vi "IV.vi"(1 "Wait for continue":bool, 2 "Run uninterrupted?":bool, 3 "Device Category IN:":string(combo)="Short Strip" caption="Device Category:", 4 "Batch No. IN:":string caption="Batch No.:", 5 "Wafer No. IN:":string caption="Wafer:", 6 "DB Serial No. IN:":string caption="DB Serial No.:") -> (0 "Done!":bool)   [LabVIEW 2018]
doc: "Performs IV measurements according to ATLAS ITk Quality Control Specifications."
uses:
  general_VIs/globals/QC_MeasurementSetup.vi
  general_VIs/globals/QC_RunInformation.vi
  InstrControl/InstrumentSetup.vi
  InstrControl/Switching/Switching.lvclass
  InstrControl/SupplyControl/SupplyControl.lvclass
  InstrControl/ArduinoControl/ArduinoControl.lvclass
  InstrControl/InstrControl.lvclass
panel:
  out "Tab Control 2":enum32{"IV Setup", "IV Scan"}(tab)
  in  "V_breakdown limit [V]":dbl=-500.0
  in  "Set current limit?":bool
  in  "Current Limit [µA]":dbl=1.0 min=0.0001 format="%.3f"
  in  "Measurement Configurations":bool
  in  "hold steps IN":i32=6 caption="hold steps"
  in  "Initial volts [V] IN":dbl caption="Initial volts [V]"
  in  "Final volts [V] IN":dbl=-700.0 caption="Final volts [V]"
  in  "step [V] IN":dbl=10.0 caption="step [V]" format="%.1f"
  in  "step interval [s] IN":i32=10 caption="step interval [s]"
  in  "Continue":bool
  in  "Quit":bool
  out "hold steps":i32=6
  out "RH":dbl[](array[numeric]) caption="RH [%]" format="%#.2f"
  out "Temp.":dbl[](array[numeric]) caption="Temp. [°C]" format="%#.2f"
  out "Current":dbl[](array[numeric]) caption="Current [nA]"
  out "Volts":dbl[](array[numeric]) caption="Volts [V]"
  out "step interval [s]":i32=10
  out "step [V]":dbl=10.0 format="%.1f"
  out "Final volts [V]":dbl=-700.0 format="%.1f"
  out "Initial volts [V]":dbl format="%.1f"
  out "Igraph":cluster{dbl[], dbl[]}(graph)
  in  "Scales":T1(ring)
  in  "Iscale":enum16{"nanoAmps", "microAmps", "milliAmps"}(ring)
  out "positive ramp?":bool
  out "Tab Control":enum32{"IV Setup", "IV Scan"}(tab)
  in  "Comments":string caption="Comments:"
  in  "Auto save files":bool=TRUE
  in  "Hardware Configurations":bool
  in  "User:":string(combo)="Vera"
  in  "IV Supply":string(combo)="Keithley 2410"
  in  "Temperature":enum16{"Read Arduino", "Enter manually"}(ring)
  in  "Manufacturer:":string(combo)="Hamamatsu"
  in  "abort":bool
  out "Device Category:":string
  out "DB Serial No.:":string
  out "Current Volts:":dbl format="%.2f"
  in  "quit (no save)":bool
  in  "Quit & Save":bool
  out "Bias On/Off:":bool
  out "STATUS 1":string
  out "Initiated:":string
  out "Wafer:":string
  out "No of steps":u32
  out "Current reading No.":u32
  out "Last reading at:":string
  # "University of\nCambridge"
  # "Strip Sensor QC: IV"
  # "Vertical Scale:"
  # "Measurement Configuration"
  # "IV Scan parameters:"
  # "Last 5 readings:"
  # "n-4"
  # "n-3"
  # "n-2"
  # "n-1"
  # "n"
  # "DUT Description"
  # "Hardware"
  # "DUT & Test Description:"
  # "Current status:"
  # "Rdg No:"
  # "out of"
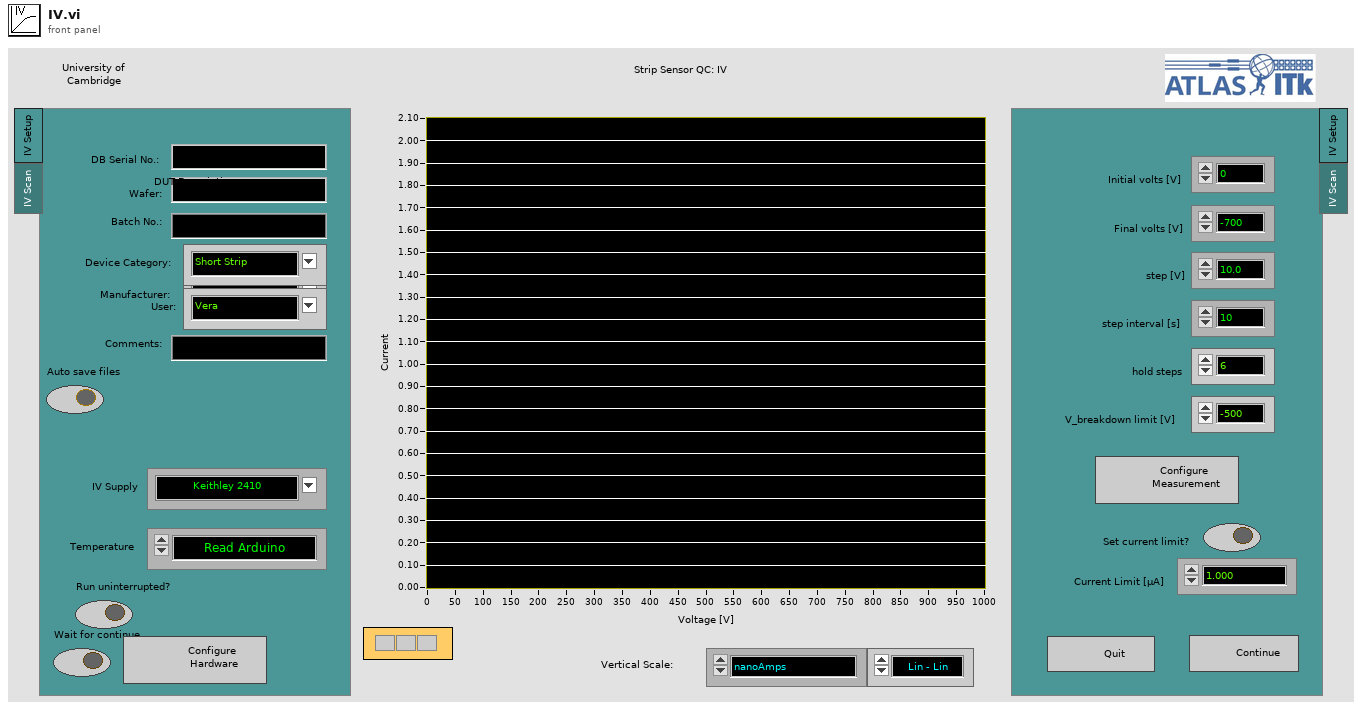
[diagram p1: front panel]
types:
  T1 = enum16{"Lin - Lin", "Log - Lin", "Lin - Log", "Log - log"}
  T2 = enum16{"Supply", "LCR", "Multimeter", "Switching"}
  T3 = enum16{"Reset", "Read Array", "Read Element", "Write Element", "Write Array", "Add Element", "Add Array"}
  T4 = enum16{"Reset", "Ground", "Striptest SMU", "Striptest LCR", "IV", "CV", "Interstrip Cap", "Interstrip Res"}
  T5 = enum32{"IV", "CV", "Stability", "Striptest", "Cis", "Ris", "PTP"}
  T6 = cluster{"Sensor Serial No.:":string, "Wafer:":string, "Batch:":string, "Manufacturer:":string, "Device Category:":string, "Database Serial No.:":string, "Date Initiated:":string, "Time Initiated:":string, "Test":string, "Probeplan used:":string, "End of Run comment:":string, "User:":string, "Vbias SMU":string, "LCR":string, "Test SMU":string, "Test DMM":string, "Comments":string}
  T7 = cluster{"Institute":string, "Manufacturers":string[], "Devices":string[], "Serialnumbers Lookup DB":string, "Data directory":string, "Backup & screenshot directory":string, "List of known users":string[], "Measurement switch not used":bool, "Measurement Switch":string, "DUT Switch":string, "Rseries IV [MOhm]":string, "Rshunt IV [MOhm]":string, "Rseries CV [MOhm]":string, "DC blocking Cap [µF]":string, "Rseries LCR [MOhm]":string, "Rseries stability [MOhm]":string, "Rshunt stability [MOhm]":string, "Rseries striptest bias [MOhm]":string, "Rseries strip pinhole [MOhm]":string}
  T8 = cluster{"Supply":refnum<class "SupplyControl.lvclass">, "Arduino":refnum<class "ArduinoControl.lvclass">, "Measurement switch":refnum<class "Switching.lvclass">, "Initial Voltage [V]":dbl, "Final Voltage [V]":dbl, "Step Size [V]":dbl, "Step Interval [s]":i32, "Number Of Steps":u32, "Ramp down steps [V]":dbl, "Ramp down Interval [s]":i32, "hold steps":i32, "Set Current Limit?":bool, "Current Limit [µA]":dbl, "Temperature Readout":enum16{"Read Arduino", "Enter manually"}, "Supply Name":string, "V_breakdown Limit [V]":dbl, "Measurement switch used?":bool}
  T9 = cluster{"VISA address":refnum<visa-resource-name>, "T sensor":enum16{"SHT", "DS"}, "Arduino":refnum<class "ArduinoControl.lvclass">}
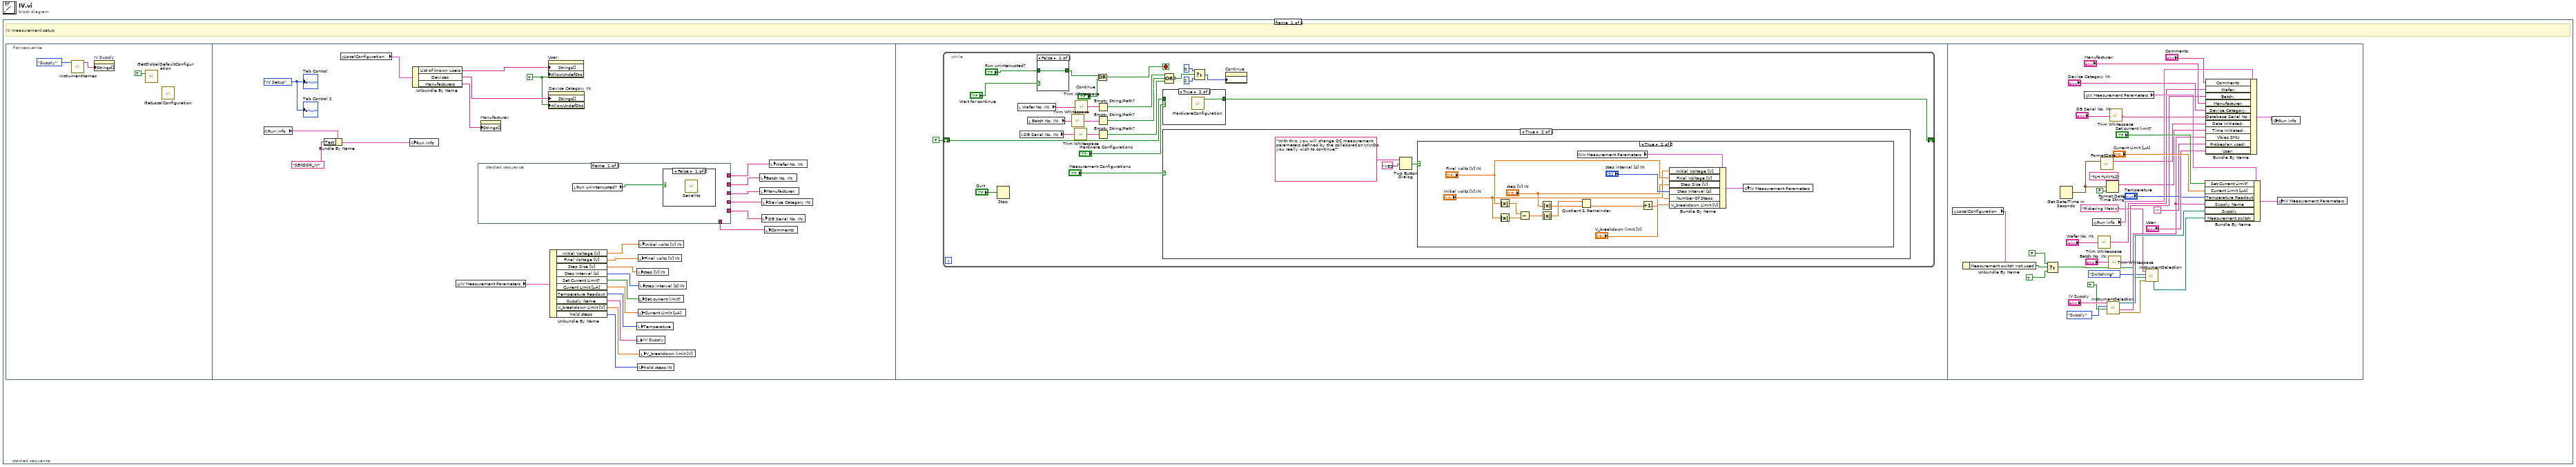
[diagram p0: block diagram]
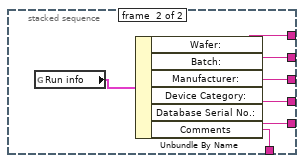
[diagram p3: hidden frame]
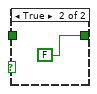
[diagram p4: hidden frame]
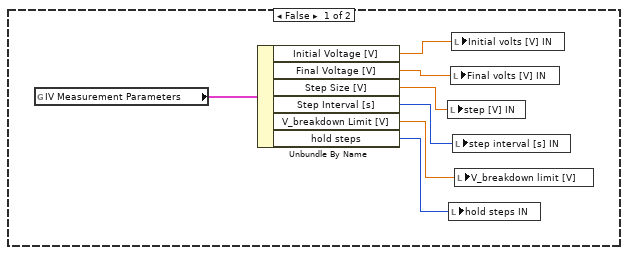
[diagram p6: hidden frame]
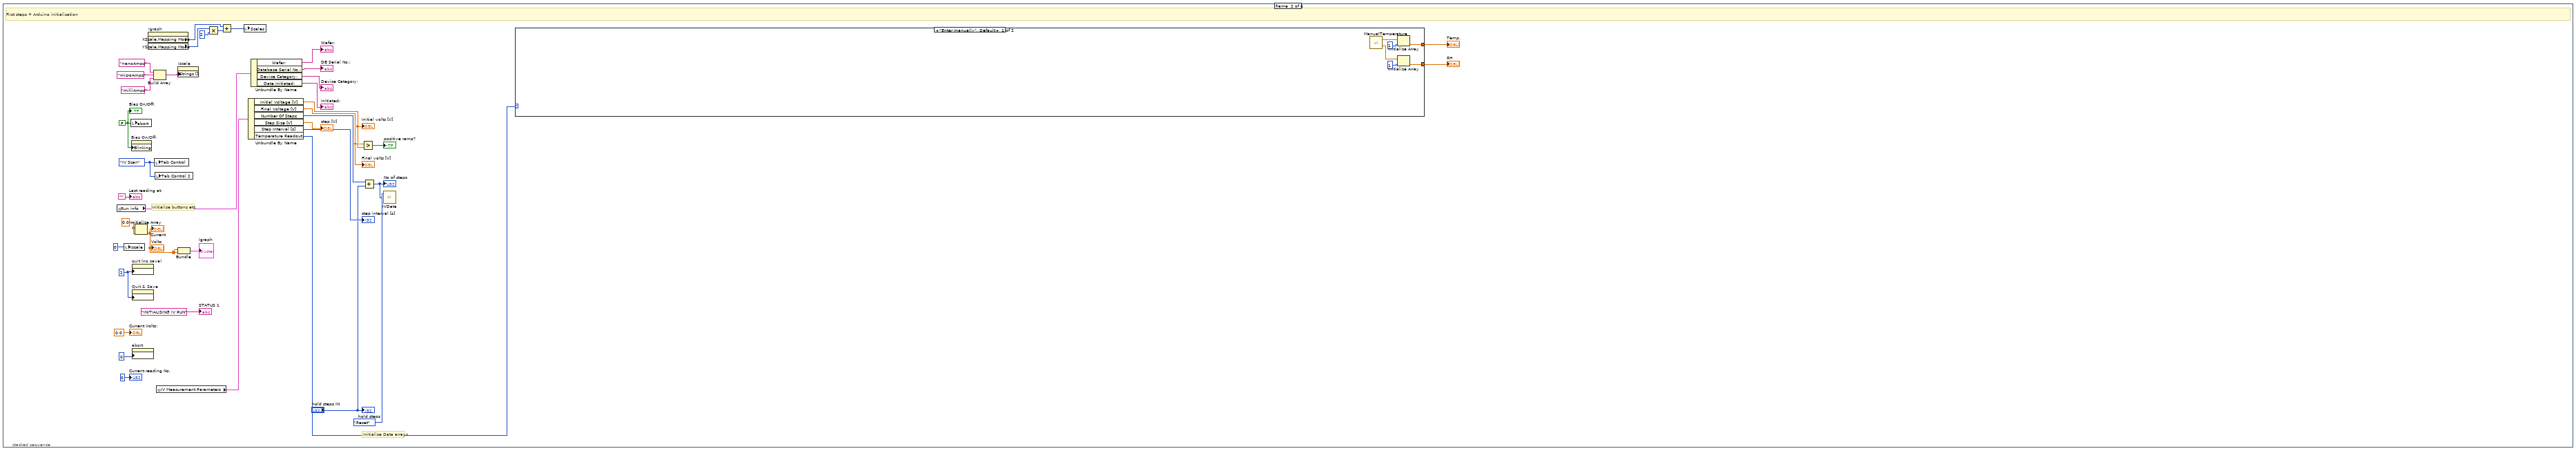
[diagram p8: hidden frame]
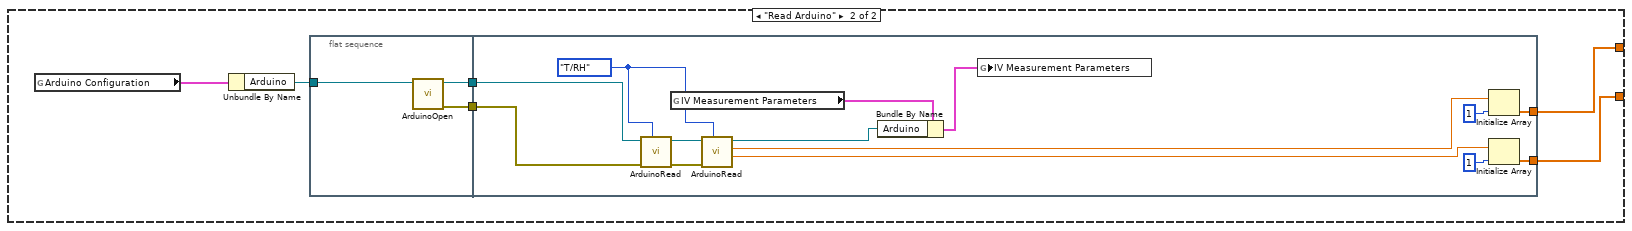
[diagram p9: hidden frame]
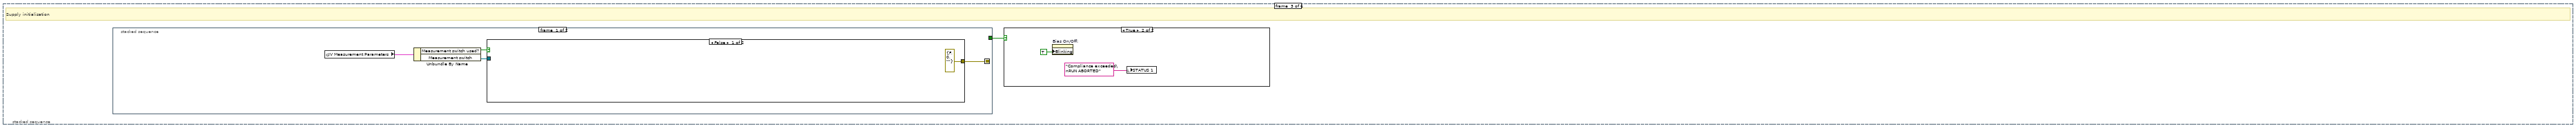
[diagram p10: hidden frame]
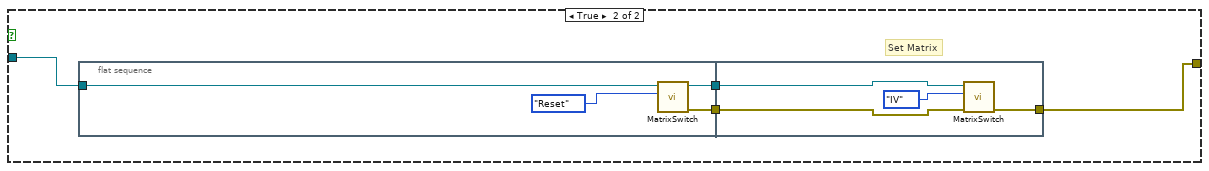
[diagram p11: hidden frame]
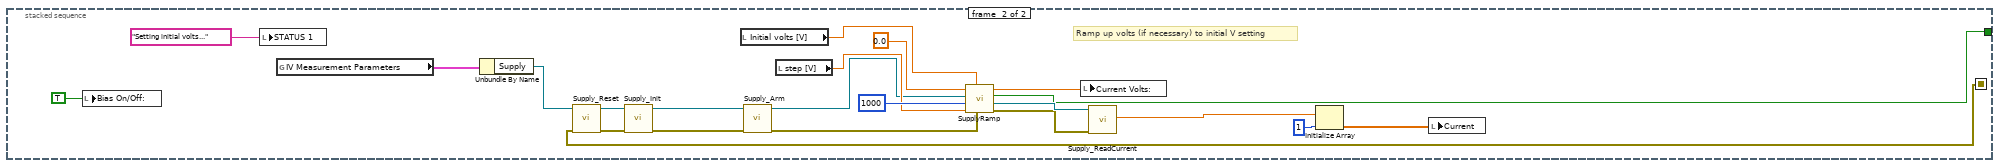
[diagram p12: hidden frame]
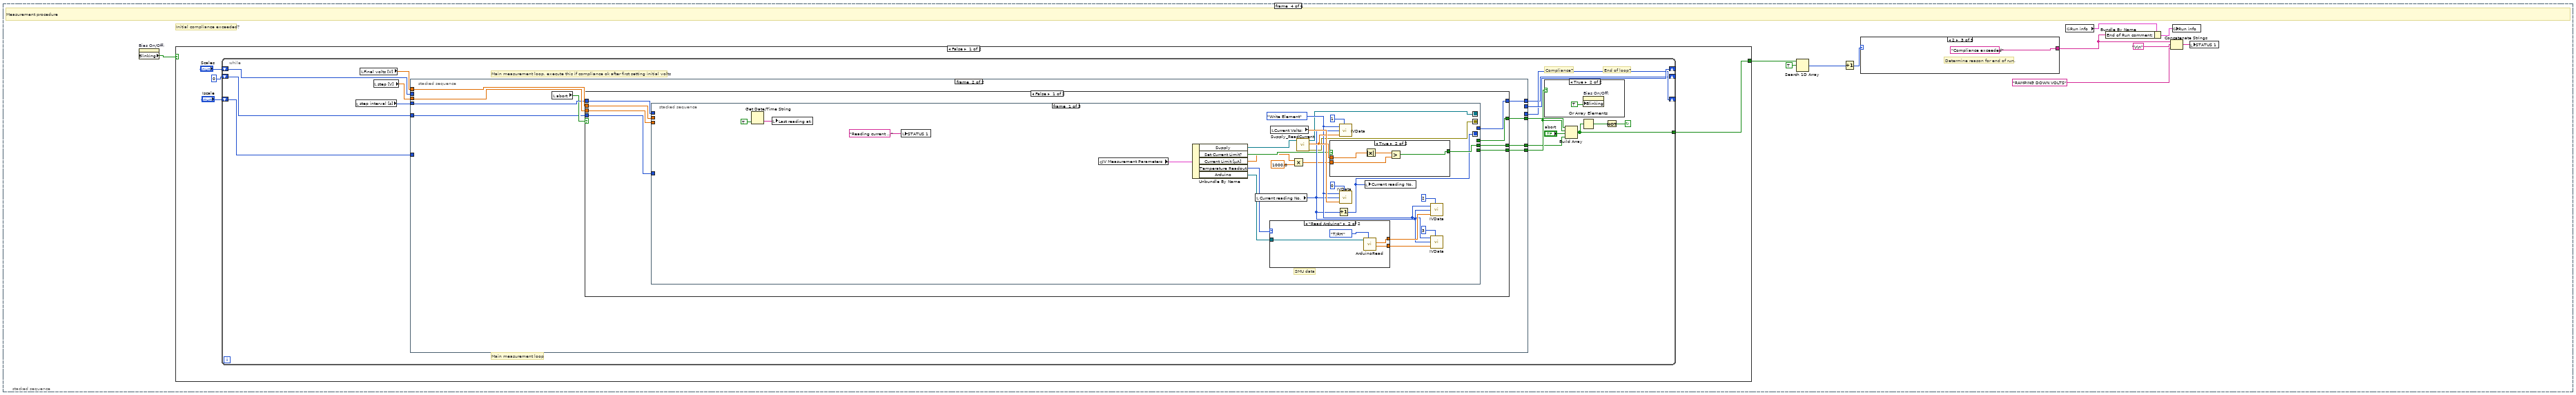
[diagram p14: hidden frame]
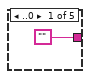
[diagram p15: hidden frame]
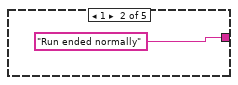
[diagram p16: hidden frame]
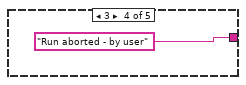
[diagram p17: hidden frame]
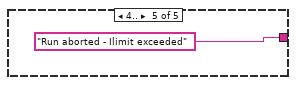
[diagram p18: hidden frame]
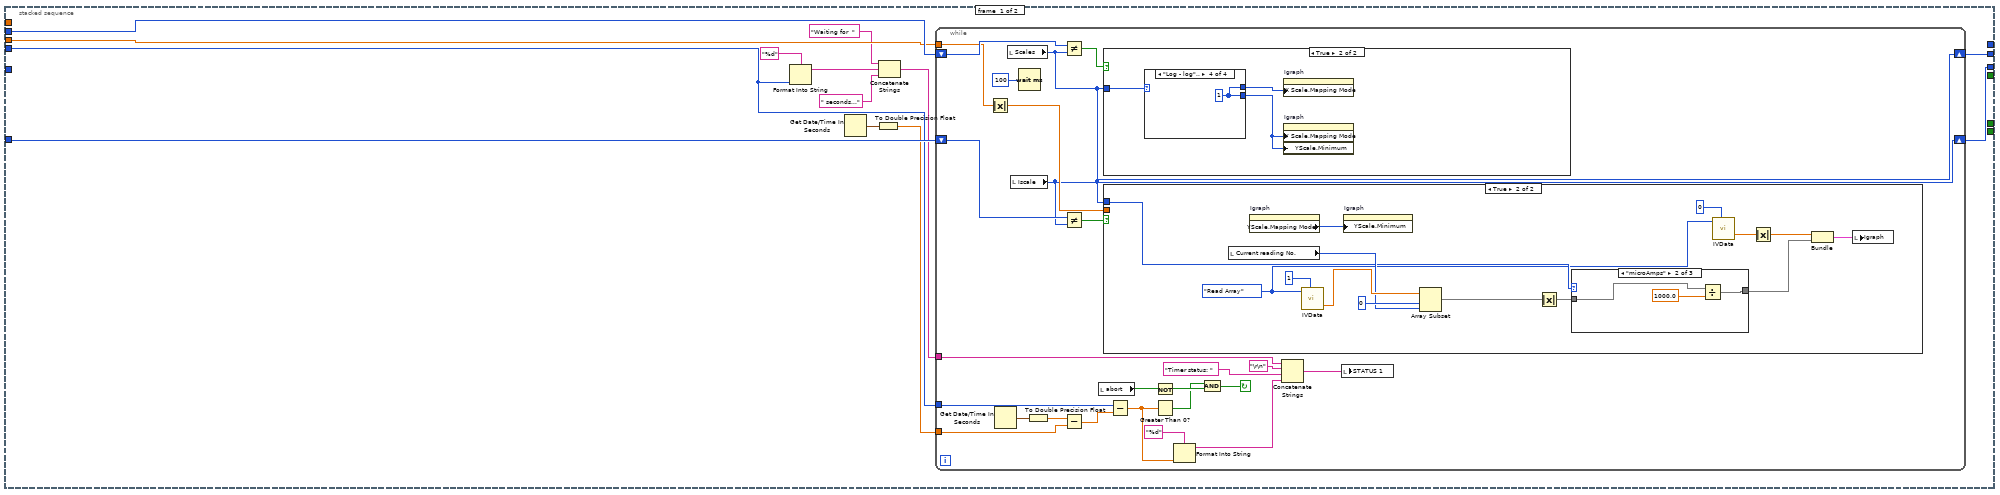
[diagram p19: hidden frame]
diagram:
  n1 = stacked-sequence {
    frame #0 {
      # "IV measurement setup"
      n2 = flat-sequence {
        frame #0 {
          n3 = call "InstrumentNames.vi"("Instrument type"=T2."Supply") -> ("Instrument names"=w2:string[])  [unwired: 9 in, 1 out]
          n4 = property on="IV Supply" class="CmbBox"("Strings[]"=w2) -> ()  [unwired: 2 in, 2 out]
          n5 = call "GetGlobalDefaultConfiguration.vi"("Read defaults?"=TRUE) -> ()  [unwired: 3 in]
          n6 = call "GetLocalConfiguration.vi"() -> ()  [unwired: 3 in, 1 out]
        }
        frame #1 {
          w11 = TRUE
          w20 = enum32{"IV Setup", "IV Scan"}."IV Setup" ("Tab Control")
          n7 = global read "QC_RunInformation.vi" "Run info"() -> (w22:T6)
          n8 = Bundle By Name(cluster=w22, "Test"="SENSOR_IV") -> (w21:T6)
          n9 = global read "QC_RunInformation.vi" "LocalConfiguration"() -> (w24:T7)
          n10 = global write "QC_RunInformation.vi" "Run info"(w21) -> ()
          n11 = Unbundle By Name(w24) -> ("List of known users"=w23:string[], "Devices"=w13:string[], "Manufacturers"=w12:string[])
          n12 = global read "QC_MeasurementSetup.vi" "IV Measurement Parameters"() -> (w27:T8)
          n13 = stacked-sequence {
            tunnel: [_ w37] -> w9
            tunnel: [_ w36] -> w8
            tunnel: [_ w35] -> w7
            tunnel: [_ w34] -> w10
            tunnel: [_ w32] -> w6
            tunnel: [_ w31] -> w4
            frame #0 {
              n14 = local read "Run uninterrupted?"() -> (w30:bool)
              n15 = case shown="False" w30 {
                frame False {
                  n16 = call "SerialNo.vi"() -> ()  [unwired: 5 in, 1 out]
                }
                frame True {
                }
              }
            }
            frame #1 {
              n17 = global read "QC_RunInformation.vi" "Run info"() -> (w33:T6)
              n18 = Unbundle By Name(w33) -> ("Wafer:"=w37:string, "Batch:"=w36:string, "Manufacturer:"=w35:string, "Device Category:"=w34:string, "Database Serial No.:"=w32:string, "Comments"=w31:string)
            }
          }
          n19 = property on="Manufacturer:" class="CmbBox"("Strings[]"=w12) -> ()  [unwired: 2 in, 2 out]
          n20 = property on="User:" class="CmbBox"("Strings[]"=w23, "AllowUndefStrs"=w11) -> ()  [unwired: 2 in, 2 out]
          n21 = property on="Device Category IN:" class="CmbBox"("Strings[]"=w13, "AllowUndefStrs"=w11) -> ()  [unwired: 2 in, 2 out]
          n22 = Unbundle By Name(w27) -> ("Initial Voltage [V]"=w18:dbl, "Final Voltage [V]"=w17:dbl, "Step Size [V]"=w16:dbl, "Step Interval [s]"=w19:i32, "Set Current Limit?"=w26:bool, "Current Limit [µA]"=w25:dbl, "Temperature Readout"=w29:enum16{"Read Arduino", "Enter manually"}, "Supply Name"=w28:string, "V_breakdown Limit [V]"=w15:dbl, "hold steps"=w14:i32)
          n23 = local write "IV Supply"(w28) -> ()
          n24 = local write "step [V] IN"(w16) -> ()
          n25 = local write "Temperature"(w29) -> ()
          n26 = local write "hold steps IN"(w14) -> ()
          n27 = local write "Final volts [V] IN"(w17) -> ()
          n28 = local write "Current Limit [µA]"(w25) -> ()
          n29 = local write "Initial volts [V] IN"(w18) -> ()
          n30 = local write "Set current limit?"(w26) -> ()
          n31 = local write "step interval [s] IN"(w19) -> ()
          n32 = local write "V_breakdown limit [V]"(w15) -> ()
          n33 = local write "Batch No. IN:"(w8) -> ()
          n34 = local write "Manufacturer:"(w7) -> ()
          n35 = local write "DB Serial No. IN:"(w6) -> ()
          n36 = local write "Device Category IN:"(w10) -> ()
          n37 = local write "Comments"(w4) -> ()
          n38 = local write "Wafer No. IN:"(w9) -> ()
          "Tab Control" <- w20
          "Tab Control 2" <- w20
        }
        frame #2 {
          n39 = while {
            shift-right: [w53] -> _
            shift-left: FALSE -> [w52]
            stop <- w50 stop-if-true
            n40 = Stop(stop? (T)="Quit") -> ()
            n41 = local read "Wafer No. IN:"() -> (w44:string)
            n42 = local read "DB Serial No. IN:"() -> (w40:string)
            n43 = local read "Batch No. IN:"() -> (w42:string)
            n44 = case shown="False" "Wait for continue" {
              tunnel: "Run uninterrupted?" -> [w62 _]
              tunnel: [w62 FALSE] -> w46
              frame False {
              }
              frame True {
              }
            }
            n45 = call <vilib>:"Trim Whitespace.vi"("string"=w42) -> ("trimmed string"=w41:string)  [unwired: 1 in]
            n46 = call <vilib>:"Trim Whitespace.vi"("string"=w40) -> ("trimmed string"=w39:string)  [unwired: 1 in]
            n47 = call <vilib>:"Trim Whitespace.vi"("string"=w44) -> ("trimmed string"=w43:string)  [unwired: 1 in]
            n48 = Or(x=w46, y="Continue") -> (x .or. y?=w50:bool)
            n49 = Empty String/Path?(string/path=w43) -> (empty?=w60:bool)
            n50 = Empty String/Path?(string/path=w41) -> (empty?=w54:bool)
            n51 = Empty String/Path?(string/path=w39) -> (empty?=w48:bool)
            n52 = case shown="True" "Hardware Configurations" {
              tunnel: [w88 w89] -> w53
              tunnel: w52 -> [w88 _]
              frame False {
              }
              frame True {
                n53 = call "HardwareConfiguration.vi"() -> ("configured?"=w89:bool)  [unwired: 11 in]
              }
            }
            n54 = case shown="True" "Measurement Configurations" {
              frame False {
              }
              frame True {
                n55 = Two Button Dialog(message="With this, you will change QC measurement parameters defined by the collaboration!\n\nDo you really wish to continue?", 2:"YES") -> (T button?=w64:bool)  [unwired: 1 in]
                n56 = case shown="True" w64 {
                  frame False {
                    n57 = global read "QC_MeasurementSetup.vi" "IV Measurement Parameters"() -> (w73:T8)
                    n58 = Unbundle By Name(w73) -> ("Initial Voltage [V]"=w71:dbl, "Final Voltage [V]"=w72:dbl, "Step Size [V]"=w70:dbl, "Step Interval [s]"=w69:i32, "V_breakdown Limit [V]"=w68:dbl, "hold steps"=w67:i32)
                    n59 = local write "step [V] IN"(w70) -> ()
                    n60 = local write "hold steps IN"(w67) -> ()
                    n61 = local write "Final volts [V] IN"(w72) -> ()
                    n62 = local write "Initial volts [V] IN"(w71) -> ()
                    n63 = local write "step interval [s] IN"(w69) -> ()
                    n64 = local write "V_breakdown limit [V]"(w68) -> ()
                  }
                  frame True {
                    n65 = Absolute Value(x="Final volts [V] IN") -> (abs(x)=w83:dbl)
                    n66 = Absolute Value(x="Initial volts [V] IN") -> (abs(x)=w82:dbl)
                    n67 = Subtract(x=w83, y=w82) -> (x-y=w77:dbl)
                    n68 = Absolute Value(x="step [V] IN") -> (abs(x)=w78:dbl)
                    n69 = Absolute Value(x=w77) -> (abs(x)=w79:dbl)
                    n70 = global read "QC_MeasurementSetup.vi" "IV Measurement Parameters"() -> (w87:T8)
                    n71 = Quotient & Remainder(x=w79, y=w78) -> (floor(x/y)=w75:dbl)  [unwired: 1 out]
                    n72 = Increment(x=w75) -> (x+1=w74:dbl)
                    n73 = Bundle By Name(cluster=w87, "Initial Voltage [V]"="Initial volts [V] IN", "Final Voltage [V]"="Final volts [V] IN", "Step Size [V]"="step [V] IN", "Step Interval [s]"="step interval [s] IN", "Number Of Steps"=w74, "V_breakdown Limit [V]"="V_breakdown limit [V]") -> (w84:T8)
                    n74 = global write "QC_MeasurementSetup.vi" "IV Measurement Parameters"(w84) -> ()
                  }
                }
              }
            }
            n75 = Compound Arithmetic op=OR(w60, w54, w48) -> (invert w59:bool)
            n76 = Select(t=0, s=w59, f=2) -> (s? t:f=w56:i32)
            n77 = property on="Continue" class="Bool"("DisabledEnum"=w56) -> ()  [unwired: 2 in, 2 out]
          }
        }
        frame #3 {
          n78 = global read "QC_RunInformation.vi" "LocalConfiguration"() -> (w106:T7)
          n79 = Unbundle By Name(w106) -> ("Measurement switch not used"=w105:bool)
          n80 = Select(t=FALSE, s=w105, f=TRUE) -> (s? t:f=w102:bool)
          n81 = Get Date/Time In Seconds() -> (seconds since 1Jan1904=w91:timestamp)
          n82 = global read "QC_MeasurementSetup.vi" "IV Measurement Parameters"() -> (w125:T8)
          n83 = global read "QC_RunInformation.vi" "Run info"() -> (w122:T6)
          n84 = call <vilib>:"Trim Whitespace.vi"("string"="Wafer No. IN:") -> ("trimmed string"=w97:string)  [unwired: 1 in]
          n85 = call "FormatDate.vi"("time stamp"=w91) -> ("Date"=w90:string)  [unwired: 1 in, 1 out]
          n86 = Format Date/Time String(time format string (%c)="%H:%M:%S", seconds (now)=w91, UTC format=FALSE) -> (date/time string=w92:string)
          n87 = call "InstrumentSelection.vi"("Verify GPIB address"=TRUE, "Instrument type"=T2."Supply", "Instrument name IN"="IV Supply") -> ("error out"=w111:errorcluster, "Instrument name OUT"=w114:string, "Supply"=w113:refnum<class "SupplyControl.lvclass">)  [unwired: 3 in, 3 out]
          n88 = call <vilib>:"Trim Whitespace.vi"("string"="Batch No. IN:") -> ("trimmed string"=w99:string)  [unwired: 1 in]
          n89 = call <vilib>:"Trim Whitespace.vi"("string"="DB Serial No. IN:") -> ("trimmed string"=w95:string)  [unwired: 1 in]
          n90 = call "InstrumentSelection.vi"("error in (no error)"=w111, "Verify GPIB address"=w102, "Instrument type"=T2."Switching", "Instrument name IN"="Pickering Matrix") -> ("Switching"=w110:refnum<class "Switching.lvclass">)  [unwired: 2 in, 5 out]
          n91 = Bundle By Name(cluster=w125, "Set Current Limit?"="Set current limit?", "Current Limit [µA]"="Current Limit [µA]", "Temperature Readout"="Temperature", "Supply Name"=w114, "Supply"=w113, "Measurement switch"=w110) -> (w126:T8)
          n92 = Bundle By Name(cluster=w122, "Comments"="Comments", "Wafer:"=w97, "Batch:"=w99, "Manufacturer:"="Manufacturer:", "Device Category:"="Device Category IN:", "Database Serial No.:"=w95, "Date Initiated:"=w90, "Time Initiated:"=w92, "Vbias SMU"=w114, "Probeplan used:"="", "User:"="User:") -> (w121:T6)
          n93 = global write "QC_RunInformation.vi" "Run info"(w121) -> ()
          n94 = global write "QC_MeasurementSetup.vi" "IV Measurement Parameters"(w126) -> ()
        }
      }
    }
    frame #1 {
      w128 = enum32{"IV Setup", "IV Scan"}."IV Scan" ("Tab Control")
      w148 = 2
      w155 = 0.0
      w147 = FALSE ("Visible")
      # "Initialise buttons etc"
      # "Initialise Data arrays"
      # "First steps + Arduino initialisation"
      n95 = global read "QC_RunInformation.vi" "Run info"() -> (w164:T6)
      n96 = local write "Iscale"(u16 0 ("Scale")) -> ()
      n97 = local write "abort"(w147) -> ()
      n98 = property on="Bias On/Off:" class="Bool (strict)"("Blinking"=w147) -> ()  [unwired: 2 in, 2 out]
      n99 = property on="quit (no save)" class="Bool"("DisabledEnum"=w148) -> ()  [unwired: 2 in, 2 out]
      n100 = property on="Quit & Save" class="Bool"("DisabledEnum"=w148) -> ()  [unwired: 2 in, 2 out]
      n101 = property on="abort" class="Bool (strict)"("DisabledEnum"=0) -> ()  [unwired: 2 in, 2 out]
      n102 = Initialize Array(w155, w155) -> (w130:dbl[])
      "Volts" <- w130
      "Current" <- w130
      n103 = property on="Igraph" class="XYGraph (strict)"() -> ("XScale.Mapping Mode"=w140:u8, "YScale.Mapping Mode"=w139:u8)  [unwired: 2 in, 2 out]
      n104 = Build Array("nanoAmps", "microAmps", "milliAmps") -> (w161:string[])
      n105 = local write "Tab Control"(w128) -> ()
      n106 = local write "Tab Control 2"(w128) -> ()
      n107 = global read "QC_MeasurementSetup.vi" "IV Measurement Parameters"() -> (w136:T8)
      n108 = property on="Iscale" class="Enum (strict)"("Strings []"=w161) -> ()  [unwired: 2 in, 2 out]
      n109 = Bundle(w130, w130) -> (→"Igraph":cluster{dbl[], dbl[]})  [unwired: 1 in]
      n110 = Multiply(x=w139, y=2) -> (x*y=w142:i32)
      n111 = Add(x=w140, y=w142) -> (x+y=w138:i32)
      n112 = local write "Scales"(w138) -> ()
      n113 = Unbundle By Name(w136) -> ("Initial Voltage [V]"=w146:dbl, "Final Voltage [V]"=w145:dbl, "Number Of Steps"=w132:u32, "Step Size [V]"=→"step [V]":dbl, "Step Interval [s]"=→"step interval [s]":i32, "Temperature Readout"=w149:enum16{"Read Arduino", "Enter manually"})
      "Initial volts [V]" <- w146
      "Final volts [V]" <- w145
      n114 = Unbundle By Name(w164) -> ("Wafer:"=→"Wafer:":string, "Database Serial No.:"=→"DB Serial No.:":string, "Device Category:"=→"Device Category:":string, "Date Initiated:"=→"Initiated:":string)
      n115 = Greater?(x=w145, y=w146) -> (0:→"positive ramp?":bool)
      n116 = Add(x=w132, y="hold steps IN") -> (x+y=w131:u32)
      "No of steps" <- w131
      n117 = call "IVData.vi"("Action"=T3."Reset", "Array Size / Index"=w131) -> ()  [unwired: 3 in, 2 out]
      n118 = case shown="\"Enter manually\", Default" w149 {
        tunnel: [w170 w177] -> w152
        tunnel: [w167 w176] -> w137
        frame "Enter manually", Default {
          n119 = call "ManualTemperature.vi"() -> ("Humidity [%] out"=w166:dbl, "Temperature [°C] out"=w171:dbl)
          n120 = Initialize Array(w171, 1) -> (w170:dbl[])
          n121 = Initialize Array(w166, 1) -> (w167:dbl[])
        }
        frame "Read Arduino" {
          n122 = global read "InstrumentSetup.vi" "Arduino Configuration"() -> (w173:T9)
          n123 = Unbundle By Name(w173) -> ("Arduino"=w172:refnum<class "ArduinoControl.lvclass">)
          n124 = flat-sequence {
            tunnel: [w178] -> w175
            tunnel: [w180] -> w174
            tunnel: w172 -> [w179]
            tunnel: [w194] -> w177
            tunnel: [w191] -> w176
            tunnel: w175 -> [w185]
            tunnel: w174 -> [w184]
            frame #0 {
              n125 = call "ArduinoOpen.vi"("ArduinoControl in"=w179) -> ("error out"=w180:errorcluster, "ArduinoControl out"=w178:refnum<class "ArduinoControl.lvclass">)  [unwired: 9 in]
            }
            frame #1 {
              w181 = enum16{"T/RH", "Interlock", "Edgesense"}."T/RH" ("Arduino function")
              n126 = call "ArduinoRead.vi"("Arduino function"=w181, "error in (no error)"=w184, "ArduinoControl in"=w185) -> ("error out"=w183:errorcluster, "ArduinoControl out"=w182:refnum<class "ArduinoControl.lvclass">)  [unwired: 3 in, 4 out]
              n127 = global read "QC_MeasurementSetup.vi" "IV Measurement Parameters"() -> (w187:T8)
              n128 = call "ArduinoRead.vi"("Arduino function"=w181, "error in (no error)"=w183, "ArduinoControl in"=w182) -> ("rel. Humidity [%]"=w189:dbl, "Temperature [°C]"=w190:dbl, "ArduinoControl out"=w188:refnum<class "ArduinoControl.lvclass">)  [unwired: 3 in, 3 out]
              n129 = Bundle By Name(cluster=w187, "Arduino"=w188) -> (w186:T8)
              n130 = global write "QC_MeasurementSetup.vi" "IV Measurement Parameters"(w186) -> ()
              n131 = Initialize Array(w190, 1) -> (w194:dbl[])
              n132 = Initialize Array(w189, 1) -> (w191:dbl[])
            }
          }
        }
      }
      "Temp." <- w152
      "RH" <- w137
      "STATUS 1" <- "INITIALISING IV RUN"
      "Bias On/Off:" <- w147
      "Last reading at:" <- ""
      "Current reading No." <- u32 0 ("Current reading No.")
      "Current Volts:" <- 0.0 ("Current Volts:")
      "hold steps" <- "hold steps IN"
    }
    frame #2 {
      # "Supply initialisation"
      n133 = stacked-sequence {
        seq-local: [w197 _] -> [_ w213]
        tunnel: [_ w214] -> w195
        frame #0 {
          n134 = global read "QC_MeasurementSetup.vi" "IV Measurement Parameters"() -> (w196:T8)
          n135 = Unbundle By Name(w196) -> ("Measurement switch used?"=w199:bool, "Measurement switch"=w198:refnum<class "Switching.lvclass">)
          n136 = case shown="False" w199 {
            tunnel: w198 -> [_ w201]
            tunnel: [errorcluster {"status"=FALSE, "code"=0, "source"=""} ("error constant") w202] -> w197
            frame False {
            }
            frame True {
              # "Set Matrix"
              n137 = flat-sequence {
                tunnel: [w208] -> w204
                tunnel: [w207] -> w203
                tunnel: w201 -> [w205]
                tunnel: w204 -> [w212]
                tunnel: w203 -> [w211]
                tunnel: [w210] -> w202
                frame #0 {
                  n138 = call-dynamic "MatrixSwitch.vi"("Action"=T4."Reset", "Switching in"=w205) -> ("error out"=w208:errorcluster, "Switching out"=w207:refnum<class "Switching.lvclass">)  [unwired: 7 in, 1 out]
                }
                frame #1 {
                  n139 = call-dynamic "MatrixSwitch.vi"("error in (no error)"=w212, "Action"=T4."IV", "Switching in"=w211) -> ("error out"=w210:errorcluster)  [unwired: 6 in, 2 out]
                }
              }
            }
          }
        }
        frame #1 {
          # "Ramp up volts (if necessary) to initial V setting"
          n140 = local write "Bias On/Off:"(TRUE ("Compliance?")) -> ()
          n141 = local write "STATUS 1"("Setting initial volts..." ("STATUS 1")) -> ()
          n142 = global read "QC_MeasurementSetup.vi" "IV Measurement Parameters"() -> (w230:T8)
          n143 = Unbundle By Name(w230) -> ("Supply"=w227:refnum<class "SupplyControl.lvclass">)
          n144 = call-dynamic "Supply_Reset.vi"("error in (no error)"=w213, "SupplyControl in"=w227) -> ("error out"=w232:errorcluster, "SupplyControl out"=w234:refnum<class "SupplyControl.lvclass">)  [unwired: 8 in]
          n145 = call-dynamic "Supply_Init.vi"("error in (no error)"=w232, "SupplyControl in"=w234) -> ("error out"=w231:errorcluster, "SupplyControl out"=w233:refnum<class "SupplyControl.lvclass">)  [unwired: 8 in]
          n146 = local read "Initial volts [V]"() -> (w222:dbl)
          n147 = call-dynamic "Supply_Arm.vi"("error in (no error)"=w231, "SupplyControl in"=w233) -> ("error out"=w220:errorcluster, "SupplyControl out"=w221:refnum<class "SupplyControl.lvclass">)  [unwired: 8 in]
          n148 = local read "step [V]"() -> (w223:dbl)
          n149 = call "SupplyRamp.vi"("error in"=w220, "Requested Voltage"=w222, "Step Size"=w223, "Step Delay"=1000, "Supply IN"=w221, "Starting Voltage"=0.0) -> ("error out"=w215:errorcluster, "Supply OUT"=w216:refnum<class "SupplyControl.lvclass">, "Compliance exceeded"=w214:bool, "Current Voltage"=w226:dbl)  [unwired: 2 in]
          n150 = local write "Current Volts:"(w226) -> ()
          n151 = call-dynamic "Supply_ReadCurrent.vi"("error in (no error)"=w215, "SupplyControl in"=w216) -> ("Current in nA"=w218:dbl)  [unwired: 7 in, 2 out]
          n152 = Initialize Array(w218, 1) -> (w217:dbl[])
          n153 = local write "Current"(w217) -> ()
        }
      }
      n154 = case shown="True" w195 {
        frame False {
        }
        frame True {
          n155 = property on="Bias On/Off:" class="Bool (strict)"("Blinking"=TRUE) -> ()  [unwired: 2 in, 2 out]
          n156 = local write "STATUS 1"("Compliance exceeded\nRUN ABORTED") -> ()
        }
      }
    }
    frame #3 {
      # "Initial compliance exceeded?"
      # "Measurement procedure"
      n157 = property on="Bias On/Off:" class="Bool (strict)"() -> ("Blinking"=w247:bool)  [unwired: 2 in, 2 out]
      n158 = case shown="False" w247 {
        tunnel: [w256 w506] -> w246
        frame False {
          n159 = while {
            shift-left: "Iscale" -> [w268]
            shift-right: [w267] -> _
            shift-left: "Scales" -> [w269]
            shift-right: [w270] -> _
            tunnel: [w266] -> w256
            shift-right: [w258] -> _
            shift-left: 0 -> [w259]
            stop <- w271 continue-if-true
            # "Main measurement loop"
            # "End of loop?"
            # "Compliance?"
            # "Main measurement loop. execute this if compliance ok after first setting initial volts"
            n160 = local read "step interval [s]"() -> (w263:i32)
            n161 = local read "Final volts [V]"() -> (w264:dbl)
            n162 = local read "step [V]"() -> (w265:dbl)
            n163 = stacked-sequence {
              tunnel: [w285 _] -> w270
              tunnel: w265 -> [w282 w349]
              tunnel: [_ w348] -> w261
              tunnel: w264 -> [_ w347]
              tunnel: w263 -> [w273 w346]
              tunnel: [_ w345] -> w262
              tunnel: w269 -> [w284 _]
              tunnel: w268 -> [w283 _]
              tunnel: [w281 _] -> w267
              tunnel: [_ w343] -> w257
              tunnel: w259 -> [_ w342]
              tunnel: [_ w341] -> w258
              frame #0 {
                n164 = Format Into String(format string="%d", w273) -> (resulting string=w278:string)  [unwired: 2 in, 1 out]
                n165 = Get Date/Time In Seconds() -> (seconds since 1Jan1904=w275:timestamp)
                n166 = To Double Precision Float(number=w275) -> (double precision float=w276:dbl)
                n167 = Concatenate Strings("Waiting for  ", w278, " seconds...") -> (w274:string)
                n168 = while {
                  tunnel: w282 -> [w294]
                  shift-left: w283 -> [w298]
                  shift-right: [w291] -> w281
                  shift-left: w284 -> [w299]
                  shift-right: [w300] -> w285
                  tunnel: w274 -> [w292]
                  tunnel: w273 -> [w304]
                  tunnel: w276 -> [w305]
                  stop <- w306 continue-if-true
                  n169 = Absolute Value(x=w294) -> (abs(x)=w293:dbl)
                  n170 = Get Date/Time In Seconds() -> (seconds since 1Jan1904=w290:timestamp)
                  n171 = local read "Scales"() -> (w300:T1)
                  n172 = local read "Iscale"() -> (w291:enum16{"nanoAmps", "microAmps", "milliAmps"})
                  n173 = Wait (ms)(milliseconds to wait=u32 100) -> ()  [unwired: 1 out]
                  n174 = To Double Precision Float(number=w290) -> (double precision float=w310:dbl)
                  n175 = Not Equal?(x=w299, y=w300) -> (x != y?=w301:bool)
                  n176 = Not Equal?(x=w298, y=w291) -> (x != y?=w289:bool)
                  n177 = Subtract(x=w310, y=w305) -> (x-y=w287:dbl)
                  n178 = local read "abort"() -> (w303:bool)
                  n179 = case shown="True" w301 {
                    tunnel: w300 -> [_ w334]
                    frame False {
                    }
                    frame True {
                      n180 = case shown="\"Log - log\".." w334 {
                        tunnel: [w335 1 0 w340] -> w333
                        tunnel: [w335 0 1 w340] -> w332
                        frame .."Lin - Lin" {
                          w335 = 0
                        }
                        frame "Log - Lin" {
                        }
                        frame "Lin - Log" {
                        }
                        frame "Log - log".. {
                          w340 = 1
                        }
                      }
                      n181 = property on="Igraph" class="XYGraph (strict)"("X Scale.Mapping Mode"=w333) -> ()  [unwired: 2 in, 2 out]
                      n182 = property on="Igraph" class="XYGraph (strict)"("Y Scale.Mapping Mode"=w332, "YScale.Minimum"=w332) -> ()  [unwired: 2 in, 2 out]
                    }
                  }
                  n183 = case shown="True" w289 {
                    tunnel: w293 -> [_ _]
                    tunnel: w291 -> [_ w319]
                    frame False {
                    }
                    frame True {
                      w313 = T3."Read Array" ("Action")
                      n184 = local read "Current reading No."() -> (w321:u32)
                      n185 = property on="Igraph" class="XYGraph (strict)"() -> ("YScale.Mapping Mode"=w315:u8)  [unwired: 2 in, 2 out]
                      n186 = call "IVData.vi"("Action"=w313, "Array No."=u32 1 ("Action")) -> ("Array OUT"=w322:dbl[])  [unwired: 3 in, 1 out]
                      n187 = property on="Igraph" class="XYGraph (strict)"("YScale.Minimum"=w315) -> ()  [unwired: 2 in, 2 out]
                      n188 = Array Subset(array=w322, index=0, length=w321) -> (w318:dbl[])
                      n189 = Absolute Value(x=w318) -> (abs(x)=w317:dbl[])
                      n190 = case shown="\"microAmps\"" w319 {
                        tunnel: [w325 w326 w330] -> w324
                        tunnel: w317 -> [w325 w328 w331]
                        frame .."nanoAmps" {
                        }
                        frame "microAmps" {
                          n191 = Divide(x=w328, y=1000.0) -> (x/y=w326:dbl[])
                        }
                        frame "milliAmps".. {
                          n192 = Divide(x=w331, y=1000000.0) -> (x/y=w330:dbl[])
                        }
                      }
                      n193 = call "IVData.vi"("Action"=w313, "Array No."=u32 0 ("Action")) -> ("Array OUT"=w312:dbl[])  [unwired: 3 in, 1 out]
                      n194 = Absolute Value(x=w312) -> (abs(x)=w311:dbl[])
                      n195 = Bundle(w311, w324) -> (w320:cluster{dbl[], dbl[]})  [unwired: 1 in]
                      n196 = local write "Igraph"(w320) -> ()
                    }
                  }
                  n197 = Subtract(x=w304, y=w287) -> (x-y=w286:dbl)
                  n198 = Not(x=w303) -> (.not. x?=w309:bool)
                  n199 = Greater Than 0?(x=w286) -> (x > 0?=w288:bool)
                  n200 = Format Into String(format string="%d", w286) -> (resulting string=w308:string)  [unwired: 2 in, 1 out]
                  n201 = And(x=w288, y=w309) -> (x .and. y?=w306:bool)
                  n202 = Concatenate Strings(w292, "\r\n", "Timer status: ", w308) -> (w302:string)
                  n203 = local write "STATUS 1"(w302) -> ()
                }
              }
              frame #1 {
                n204 = local read "abort"() -> (w344:bool)
                n205 = case shown="False" w344 {
                  tunnel: [w357 w503] -> w345
                  tunnel: w346 -> [w356 _]
                  tunnel: w347 -> [w355 _]
                  tunnel: [w353 w503] -> w348
                  tunnel: w349 -> [w354 _]
                  tunnel: [w352 w503] -> w343
                  tunnel: w342 -> [w351 w502]
                  tunnel: [w350 w502] -> w341
                  frame False {
                    n206 = stacked-sequence {
                      seq-local: [w372 _ _] -> [_ w407 _]
                      seq-local: [w367 _ _] -> [_ _ w467]
                      seq-local: [w366 _ _] -> [_ _ w468]
                      tunnel: w354 -> [_ w404 w473]
                      tunnel: w355 -> [_ _ w465]
                      tunnel: [_ _ w471] -> w357
                      tunnel: [_ _ w470] -> w353
                      tunnel: w356 -> [_ _ _]
                      tunnel: [w376 _ _] -> w352
                      tunnel: w351 -> [_ w405 w459]
                      tunnel: [_ _ w458] -> w350
                      frame #0 {
                        w370 = T3."Write Element" ("Action")
                        # "SMU data"
                        n207 = Get Date/Time String(want seconds? (F)=TRUE) -> (time string=w373:string)  [unwired: 2 in, 1 out]
                        n208 = local write "Last reading at:"(w373) -> ()
                        n209 = local write "STATUS 1"("Reading current ..." ("status")) -> ()
                        n210 = global read "QC_MeasurementSetup.vi" "IV Measurement Parameters"() -> (w365:T8)
                        n211 = Unbundle By Name(w365) -> ("Supply"=w359:refnum<class "SupplyControl.lvclass">, "Set Current Limit?"=w364:bool, "Current Limit [µA]"=w361:dbl, "Temperature Readout"=w363:enum16{"Read Arduino", "Enter manually"}, "Arduino"=w358:refnum<class "ArduinoControl.lvclass">)
                        n212 = local read "Current reading No."() -> (w369:u32)
                        n213 = case shown="\"Read Arduino\"" w363 {
                          tunnel: [w386 w392] -> w374
                          tunnel: [w383 w391] -> w368
                          tunnel: w358 -> [_ w390]
                          frame "Enter manually", Default {
                            n214 = local read "Temp."() -> (w388:dbl[])
                            n215 = local read "RH"() -> (w384:dbl[])
                            n216 = Index Array(array=w388, index=0) -> (element=w386:dbl)
                            n217 = Index Array(array=w384, index=0) -> (element=w383:dbl)
                          }
                          frame "Read Arduino" {
                            n218 = call "ArduinoRead.vi"("Arduino function"=enum16{"T/RH", "Interlock", "Edgesense"}."T/RH", "ArduinoControl in"=w390) -> ("rel. Humidity [%]"=w391:dbl, "Temperature [°C]"=w392:dbl)  [unwired: 4 in, 4 out]
                          }
                        }
                        n219 = local read "Current Volts:"() -> (w378:dbl)
                        n220 = Multiply(x=w361, y=1000.0) -> (x*y=w360:dbl)
                        n221 = call-dynamic "Supply_ReadCurrent.vi"("SupplyControl in"=w359) -> ("error out"=w366:errorcluster, "Current in nA"=w377:dbl, "SupplyControl out"=w367:refnum<class "SupplyControl.lvclass">)  [unwired: 8 in]
                        n222 = case shown="True" w364 {
                          tunnel: w377 -> [_ w397]
                          tunnel: w360 -> [_ w395]
                          tunnel: [FALSE w394] -> w376
                          frame False {
                          }
                          frame True {
                            n223 = Absolute Value(x=w397) -> (abs(x)=w396:dbl)
                            n224 = Greater?(x=w396, y=w395) -> (0:w394:bool)
                          }
                        }
                        n225 = Increment(x=w369) -> (x+1=w372:u32)
                        n226 = call "IVData.vi"("Action"=w370, "Array No."=u32 1, "Array Size / Index"=w369, "Data IN"=w377) -> ()  [unwired: 1 in, 2 out]
                        n227 = call "IVData.vi"("Action"=w370, "Array No."=0, "Array Size / Index"=w369, "Data IN"=w378) -> ()  [unwired: 1 in, 2 out]
                        n228 = local write "Current reading No."(w372) -> ()
                        n229 = call "IVData.vi"("Action"=w370, "Array No."=u32 2, "Array Size / Index"=w369, "Data IN"=w374) -> ()  [unwired: 1 in, 2 out]
                        n230 = call "IVData.vi"("Action"=w370, "Array No."=u32 3, "Array Size / Index"=w369, "Data IN"=w368) -> ()  [unwired: 1 in, 2 out]
                      }
                      frame #1 {
                        w400 = T3."Read Array" ("Action")
                        w417 = u32 5 ("y")
                        # "Update plots"
                        n231 = Greater Than 0?(x=w405) -> (x > 0?=w406:bool)
                        n232 = property on="Igraph" class="XYGraph (strict)"() -> ("YScale.Mapping Mode"=w408:u8)  [unwired: 2 in, 2 out]
                        n233 = Select(t=0.01, s=w406, f=w404) -> (s? t:f=w403:dbl)
                        n234 = property on="Igraph" class="XYGraph (strict)"("YScale.Minimum"=w408) -> ()  [unwired: 2 in, 2 out]
                        n235 = call "IVData.vi"("Action"=w400, "Array No."=1) -> ("Array OUT"=w419:dbl[])  [unwired: 3 in, 1 out]
                        n236 = Absolute Value(x=w403) -> ()  [unwired: 1 out]
                        n237 = Greater?(x=w407, y=w417) -> (0:w416:bool)
                        n238 = case shown="True" w416 {
                          tunnel: w407 -> [w423 w426]
                          tunnel: w417 -> [_ w425]
                          tunnel: [w423 w425] -> w415
                          tunnel: [0 w424] -> w413
                          frame False {
                          }
                          frame True {
                            n239 = Subtract(x=w426, y=w425) -> (x-y=w424:u32)
                          }
                        }
                        n240 = Array Subset(array=w419, index=0, length=w407) -> (w412:dbl[])
                        n241 = local read "Iscale"() -> (w418:enum16{"nanoAmps", "microAmps", "milliAmps"})
                        n242 = Absolute Value(x=w412) -> (abs(x)=w411:dbl[])
                        n243 = case shown="\"microAmps\"" w418 {
                          tunnel: [w451 w452 w455] -> w421
                          tunnel: w411 -> [w451 w454 w457]
                          frame .."nanoAmps" {
                          }
                          frame "microAmps" {
                            n244 = Divide(x=w454, y=1000.0) -> (x/y=w452:dbl[])
                          }
                          frame "milliAmps".. {
                            n245 = Divide(x=w457, y=1000000.0) -> (x/y=w455:dbl[])
                          }
                        }
                        n246 = call "IVData.vi"("Action"=w400, "Array No."=0) -> ("Array OUT"=w399:dbl[])  [unwired: 3 in, 1 out]
                        n247 = Absolute Value(x=w399) -> (abs(x)=w398:dbl[])
                        n248 = for {
                          N: 4 -> [_]
                          tunnel: w415 -> [w431]
                          tunnel: w413 -> [w430]
                          tunnel: w407 -> [w427]
                          i -> [w432]
                          n249 = call "IVData.vi"("Action"=T3."Read Array", "Array No."=w432) -> ("Array OUT"=w429:dbl[])  [unwired: 3 in, 1 out]
                          n250 = case shown="2" w432 {
                            tunnel: w431 -> [w435 w439 _ _]
                            tunnel: w430 -> [w436 w440 _ _]
                            tunnel: w429 -> [w434 w438 w444 w449]
                            tunnel: w427 -> [_ _ w442 w447]
                            frame ..0 {
                              n251 = Array Subset(array=w434, index=w436, length=w435) -> (w433:dbl[])
                              n252 = local write "Volts"(w433) -> ()
                            }
                            frame 1 {
                              n253 = Array Subset(array=w438, index=w440, length=w439) -> (w437:dbl[])
                              n254 = local write "Current"(w437) -> ()
                            }
                            frame 2 {
                              n255 = Decrement(x=w442) -> (x-1=w441:u32)
                              n256 = Array Subset(array=w444, index=w441, length=1) -> (w443:dbl[])
                              n257 = local write "Temp."(w443) -> ()
                            }
                            frame 3.. {
                              n258 = Decrement(x=w447) -> (x-1=w446:u32)
                              n259 = Array Subset(array=w449, index=w446, length=1) -> (w448:dbl[])
                              n260 = local write "RH"(w448) -> ()
                            }
                          }
                        }
                        n261 = Bundle(w398, w421) -> (w409:cluster{dbl[], dbl[]})  [unwired: 1 in]
                        n262 = local write "Igraph"(w409) -> ()
                      }
                      frame #2 {
                        # "Increment volts and check for end of loop"
                        n263 = local read "positive ramp?"() -> (w469:bool)
                        n264 = local read "Current Volts:"() -> (w460:dbl)
                        n265 = case shown="True" w469 {
                          tunnel: w465 -> [w476 w480]
                          tunnel: w473 -> [w477 w483]
                          tunnel: [w475 w482] -> w461
                          tunnel: [w474 w479] -> w472
                          tunnel: w460 -> [w478 w481]
                          frame False {
                            n266 = Subtract(x=w478, y=w477) -> (x-y=w474:dbl)
                            n267 = Greater Or Equal?(x=w474, y=w476) -> (x >= y?=w475:bool)
                          }
                          frame True {
                            n268 = Add(x=w481, y=w483) -> (x+y=w479:dbl)
                            n269 = Less Or Equal?(x=w479, y=w480) -> (x <= y?=w482:bool)
                          }
                        }
                        n270 = Quotient & Remainder(x=w460, y=w465) -> (x-y*floor(x/y)=w466:dbl, floor(x/y)=w464:dbl)
                        n271 = Not Equal To 0?(x=w466) -> (x != 0?=w462:bool)
                        n272 = Equal To 0?(x=w464) -> (x = 0?=w463:bool)
                        n273 = Or(x=w462, y=w463) -> ()  [unwired: 1 out]
                        n274 = case shown="False" w461 {
                          tunnel: w472 -> [_ w498]
                          tunnel: [w487 FALSE] -> w471
                          tunnel: [FALSE w499] -> w470
                          tunnel: w460 -> [_ w496]
                          tunnel: w468 -> [_ w495]
                          tunnel: w467 -> [_ w494]
                          tunnel: w459 -> [w486 _]
                          tunnel: [w485 0] -> w458
                          frame False {
                            (unwired) TRUE
                            n275 = Increment(x=w486) -> (x+1=w485:i32)
                            n276 = local read "hold steps"() -> (w484:i32)
                            n277 = Greater Or Equal?(x=w486, y=w484) -> (x >= y?=w487:bool)
                          }
                          frame True {
                            n278 = local read "step [V]"() -> (w492:dbl)
                            n279 = call "SupplyRamp.vi"("error in"=w495, "Requested Voltage"=w498, "Step Size"=w492, "Step Delay"=100, "Supply IN"=w494, "Starting Voltage"=w496) -> ("error out"=w490:errorcluster, "Compliance exceeded"=w499:bool, "Current Voltage"=w493:dbl)  [unwired: 2 in, 1 out]
                            n280 = case shown="No Error" w490 {
                              tunnel: w493 -> [w501 _]
                              frame No Error {
                                n281 = local write "Current Volts:"(w501) -> ()
                              }
                              frame Error {
                              }
                            }
                            n282 = property on="Bias On/Off:" class="Bool (strict)"("Blinking"=w499) -> ()  [unwired: 2 in, 2 out]
                            n283 = local write "STATUS 1"("Incrementing volts.") -> ()
                          }
                        }
                      }
                    }
                  }
                  frame True {
                    w503 = FALSE
                  }
                }
              }
            }
            n284 = case shown="True" w261 {
              frame False {
              }
              frame True {
                n285 = property on="Bias On/Off:" class="Bool (strict)"("Blinking"=TRUE) -> ()  [unwired: 2 in, 2 out]
              }
            }
            n286 = Build Array(w262, w261, "abort", w257) -> (w266:bool[])
            n287 = Or Array Elements(Boolean array=w266) -> (logical OR=w272:bool)
            n288 = Not(x=w272) -> (.not. x?=w271:bool)
          }
        }
        frame True {
          w505 = FALSE
          # "compliance was exceeded when first voltage applied."
          # "Flag compliance as reason for end of run"
          n289 = local write "STATUS 1"("Run aborted - compliance exceeded.") -> ()
          n290 = Build Array(w505, TRUE, w505, w505) -> (w506:bool[])
        }
      }
      n291 = Search 1D Array(1D array=w246, element=TRUE) -> (index of element=w244:i32)  [unwired: 1 in]
      n292 = Increment(x=w244) -> (x+1=w243:i32)
      n293 = case shown="2" w243 {
        tunnel: ["" "Run ended normally" "Compliance exceeded" "Run aborted - by user" "Run aborted - Ilimit exceeded"] -> w238
        frame ..0 {
        }
        frame 1 {
        }
        frame 2 {
          # "Determine reason for end of run."
        }
        frame 3 {
        }
        frame 4.. {
        }
      }
      n294 = global read "QC_RunInformation.vi" "Run info"() -> (w242:T6)
      n295 = Bundle By Name(cluster=w242, "End of Run comment:"=w238) -> (w237:T6)
      n296 = Concatenate Strings(w238, "\r\n", "RAMPING DOWN VOLTS") -> (w241:string)
      n297 = global write "QC_RunInformation.vi" "Run info"(w237) -> ()
      n298 = local write "STATUS 1"(w241) -> ()
    }
    frame #4 {
      # "Ramp down and switch off supply"
      n299 = stacked-sequence {
        frame #0 {
          # "Tie up loose ends. Set volts to zero and switch to standby"
          # "Ramp down volts now"
          n300 = global read "QC_MeasurementSetup.vi" "IV Measurement Parameters"() -> (w517:T8)
          n301 = Unbundle By Name(w517) -> ("Supply"=w514:refnum<class "SupplyControl.lvclass">, "Ramp down steps [V]"=w516:dbl, "Ramp down Interval [s]"=w515:i32, "Measurement switch"=w509:refnum<class "Switching.lvclass">, "Measurement switch used?"=w510:bool)
          n302 = local read "Current Volts:"() -> (w522:dbl)
          n303 = Multiply(x=w515, y=1000) -> (x*y=w519:i32)
          n304 = call "SupplyRamp.vi"("Requested Voltage"=0.0, "Step Size"=w516, "Step Delay"=w519, "Supply IN"=w514, "Starting Voltage"=w522) -> ("error out"=w513:errorcluster, "Supply OUT"=w512:refnum<class "SupplyControl.lvclass">, "Current Voltage"=w520:dbl)  [unwired: 3 in, 1 out]
          n305 = local write "Current Volts:"(w520) -> ()
          n306 = call-dynamic "Supply_Stby.vi"("error in (no error)"=w513, "SupplyControl in"=w512) -> ("error out"=w511:errorcluster)  [unwired: 8 in, 1 out]
          n307 = case shown="True" w510 {
            tunnel: w509 -> [_ w525]
            tunnel: w511 -> [_ w524]
            frame False {
            }
            frame True {
              n308 = call-dynamic "MatrixSwitch.vi"("error in (no error)"=w524, "Action"=T4."Reset", "Switching in"=w525) -> ()  [unwired: 6 in, 3 out]
            }
          }
        }
        frame #1 {
          w530 = 0
          n309 = local write "Bias On/Off:"(FALSE ("Visible")) -> ()
          n310 = local write "Current Volts:"(0.0 ("Current Volts:")) -> ()
          n311 = property on="Quit & Save" class="Bool"("DisabledEnum"=w530) -> ()  [unwired: 2 in, 2 out]
          n312 = property on="quit (no save)" class="Bool"("DisabledEnum"=w530) -> ()  [unwired: 2 in, 2 out]
          n313 = property on="abort" class="Bool (strict)"("DisabledEnum"=2) -> ()  [unwired: 2 in, 2 out]
          n314 = local write "STATUS 1"("Run finished. \nSave data?" ("STATUS 1")) -> ()
        }
        frame #2 {
          n315 = Current VI's Path() -> (path=w532:path)
          n316 = call "SaveJPEG.vi"("Test"="IV", "File Path Control"=w532) -> ()  [unwired: 1 in, 2 out]
        }
      }
    }
    frame #5 {
      # "Loop and await decision on whether to save or junk data"
      # "Display and save data"
      n317 = local read "Scales"() -> (w545:T1)
      n318 = local read "Iscale"() -> (w544:enum16{"nanoAmps", "microAmps", "milliAmps"})
      n319 = while {
        shift-left: w544 -> [w618]
        shift-right: [w617] -> _
        shift-left: w545 -> [w620]
        shift-right: [w619] -> _
        tunnel: [w611] -> w547
        tunnel: ["quit (no save)"] -> w546
        stop <- w616 continue-if-true
        n320 = local read "Scales"() -> (w619:T1)
        n321 = local read "Iscale"() -> (w617:enum16{"nanoAmps", "microAmps", "milliAmps"})
        n322 = Not Equal?(x=w620, y=w619) -> (x != y?=w614:bool)
        n323 = Not Equal?(x=w618, y=w617) -> (x != y?=w613:bool)
        n324 = case shown="True" w614 {
          tunnel: w619 -> [_ w647]
          frame False {
          }
          frame True {
            n325 = case shown="..\"Lin - Lin\"" w647 {
              tunnel: [w648 1 0 w653] -> w646
              tunnel: [w648 0 1 w653] -> w645
              frame .."Lin - Lin" {
                w648 = 0
              }
              frame "Log - Lin" {
              }
              frame "Lin - Log" {
              }
              frame "Log - log".. {
                w653 = 1
              }
            }
            n326 = property on="Igraph" class="XYGraph (strict)"("X Scale.Mapping Mode"=w646) -> ()  [unwired: 2 in, 2 out]
            n327 = property on="Igraph" class="XYGraph (strict)"("Y Scale.Mapping Mode"=w645, "YScale.Minimum"=w645) -> ()  [unwired: 2 in, 2 out]
          }
        }
        n328 = case shown="True" w613 {
          tunnel: w617 -> [_ w633]
          frame False {
          }
          frame True {
            w626 = T3."Read Array" ("Action")
            n329 = property on="Igraph" class="XYGraph (strict)"() -> ("YScale.Mapping Mode"=w629:u8)  [unwired: 2 in, 2 out]
            n330 = property on="Igraph" class="XYGraph (strict)"("YScale.Minimum"=w629) -> ()  [unwired: 2 in, 2 out]
            n331 = global read "QC_MeasurementSetup.vi" "IV Measurement Parameters"() -> (w628:T8)
            n332 = Unbundle By Name(w628) -> ("Number Of Steps"=w625:u32)
            n333 = local read "hold steps"() -> (w624:i32)
            n334 = Add(x=w625, y=w624) -> (x+y=w623:u32)
            n335 = call "IVData.vi"("Action"=w626, "Array No."=u32 1 ("Action")) -> ("Array OUT"=w635:dbl[])  [unwired: 3 in, 1 out]
            n336 = Array Subset(array=w635, index=0, length=w623) -> (w632:dbl[])
            n337 = Absolute Value(x=w632) -> (abs(x)=w631:dbl[])
            n338 = case shown="\"microAmps\"" w633 {
              tunnel: [w638 w639 w643] -> w637
              tunnel: w631 -> [w638 w641 w644]
              frame .."nanoAmps" {
              }
              frame "microAmps" {
                n339 = Divide(x=w641, y=1000.0) -> (x/y=w639:dbl[])
              }
              frame "milliAmps".. {
                n340 = Divide(x=w644, y=1000000.0) -> (x/y=w643:dbl[])
              }
            }
            n341 = call "IVData.vi"("Action"=w626, "Array No."=u32 0 ("Action")) -> ("Array OUT"=w622:dbl[])  [unwired: 3 in, 1 out]
            n342 = Absolute Value(x=w622) -> (abs(x)=w621:dbl[])
            n343 = Bundle(w621, w637) -> (w634:cluster{dbl[], dbl[]})  [unwired: 1 in]
            n344 = local write "Igraph"(w634) -> ()
          }
        }
        n345 = local read "Run uninterrupted?"() -> (w610:bool)
        n346 = Or(x=w610, y="Auto save files") -> (x .or. y?=w608:bool)
        n347 = Select(t=w608, s=w608, f="Quit & Save") -> (s? t:f=w611:bool)
        n348 = Not Or(1:"quit (no save)", 2:w611) -> (0:w616:bool)
      }
      n349 = global read "QC_MeasurementSetup.vi" "IV Measurement Parameters"() -> (w543:T8)
      n350 = Unbundle By Name(w543) -> ("Temperature Readout"=w542:enum16{"Read Arduino", "Enter manually"}, "Arduino"=w536:refnum<class "ArduinoControl.lvclass">)
      n351 = case shown="\"Read Arduino\"" w542 {
        tunnel: w536 -> [_ w607]
        frame "Enter manually", Default {
        }
        frame "Read Arduino" {
          n352 = call "ArduinoClose.vi"("ArduinoControl in"=w607) -> ()  [unwired: 9 in, 2 out]
        }
      }
      n353 = case shown="False" w546 {
        tunnel: [FALSE w655] -> w548
        frame False {
        }
        frame True {
          n354 = Two Button Dialog(message="Are you sure you don't want to save the data?", 1:"Quit" ("F button name (\"Cancel\")"), 2:"Save data" ("T button name (\"OK\")")) -> (T button?=w655:bool)
        }
      }
      n355 = Or(x=w547, y=w548) -> (x .or. y?=w541:bool)
      n356 = flat-sequence {
        tunnel: w541 -> [w560]
        tunnel: [w560] -> w534
        tunnel: [TRUE] -> w533
        tunnel: [w605] -> w535
        tunnel: [w606] -> w537
        tunnel: w534 -> [w606]
        tunnel: w533 -> [w605]
        frame #0 {
          n357 = global read "QC_MeasurementSetup.vi" "IV Measurement Parameters"() -> (w569:T8)
          n358 = Unbundle By Name(w569) -> ("V_breakdown Limit [V]"=w564:dbl)
          n359 = call "ScanFeedback.vi"("measurement type"=T5."IV") -> ("V breakdown"=w562:dbl)  [unwired: 4 in, 4 out]
          n360 = Absolute Value(x=w562) -> (abs(x)=w561:dbl)
          n361 = Absolute Value(x=w564) -> (abs(x)=w563:dbl)
          n362 = Greater Or Equal?(x=w561, y=w563) -> (x >= y?=w565:bool)
          n363 = local read "Run uninterrupted?"() -> (w558:bool)
          n364 = local read "Auto save files"() -> (w557:bool)
          n365 = Or(x=w558, y=w557) -> (x .or. y?=w549:bool)
          n366 = case shown="True" w560 {
            tunnel: ["" w603] -> w570
            tunnel: [_ w591] -> w568
            tunnel: w549 -> [_ w576]
            tunnel: [_ w577] -> w553
            frame False {
            }
            frame True {
              w599 = T3."Read Array" ("Action")
              n367 = local write "STATUS 1"("Saving Data ...") -> ()
              n368 = call "IVData.vi"("Action"=w599, "Array No."=u32 0 ("Action")) -> ("Array OUT"=w594:dbl[])  [unwired: 3 in, 1 out]
              n369 = call "IVData.vi"("Action"=w599, "Array No."=u32 1 ("Action")) -> ("Array OUT"=w574:dbl[])  [unwired: 3 in, 1 out]
              n370 = Array Size(array=w574) -> (size(s)=w573:i32)
              n371 = call "IVData.vi"("Action"=w599, "Array No."=u32 3 ("Action")) -> ("Array OUT"=w601:dbl[])  [unwired: 3 in, 1 out]
              n372 = call "IVData.vi"("Action"=w599, "Array No."=u32 2 ("Action")) -> ("Array OUT"=w600:dbl[])  [unwired: 3 in, 1 out]
              n373 = local read "Current reading No."() -> (w585:u32)
              n374 = Initialize Array(0.0 ("element"), w573) -> (w572:dbl[])
              n375 = Build Array(w594, w574, w572) -> (w593:dbl[][])
              n376 = Add Array Elements(numeric array=w601) -> (sum=w588:dbl)
              n377 = Add Array Elements(numeric array=w600) -> (sum=w586:dbl)
              n378 = Transpose 2D Array(2D array=w593) -> (transposed array=w583:dbl[][])
              n379 = Array Size(array=w583) -> (size(s)=w582:i32[])
              n380 = Divide(x=w586, y=w585) -> (x/y=w584:dbl)
              n381 = Divide(x=w588, y=w585) -> (x/y=w587:dbl)
              n382 = Index Array(array=w582, index #1=0, index #2=1) -> (element #1=w579:i32, element #2=w578:i32)
              n383 = call "SaveDataFile.vi"("Data Array"=w583, "Temperature"=w584, "Run uninterrupted?"=w576, "Humidity"=w587, "no. of arrays"=w578, "Actual array lengths"=w579, "Array Titles"="Voltage[V] Current[nA] Shunt_voltage[mV]", "Strip Segment"="", "Arrays format"="%010.2f") -> ("Filename OUT"=w577:string, "Path + Filename OUT"=w603:string, "Error Out"=w591:errorcluster)  [unwired: 3 in, 1 out]
            }
          }
          n384 = global read "QC_RunInformation.vi" "LocalConfiguration"() -> (w556:T7)
          n385 = call "WriteLogFile.vi"("Run uninterrupted?"=w549, "Automatic warning"="", "Data File"=w570, "Error In"=w568, "DUT passed?"=w565, "Value TechSpec criteria"=w562, "Files saved?"=w560) -> ()  [unwired: 4 in, 1 out]
          n386 = Unbundle By Name(w556) -> ("Backup & screenshot directory"=w554:string)
          n387 = Search/Split String(string=w553, search string/char (-)=".dat") -> (substring before match=w551:string)  [unwired: 1 in, 2 out]
          n388 = String To Path(string=w554) -> (path=w555:path)
          n389 = control-ref of="This VI"() -> (w550:refnum<vi>)
          n390 = call "CreateScreenShot.vi"("Screenshot name"=w551, "base path"=w555, "reference"=w550) -> ()  [unwired: 8 in, 1 out]
        }
        frame #1 {
          w604 = FALSE
          n391 = local write "Wait for continue"(w604) -> ()
          n392 = local write "Run uninterrupted?"(w604) -> ()
        }
      }
      n393 = Select(t="Run finished.\nData saved." ("STATUS 1"), s=w537, f="Run finished.\nData not saved." ("STATUS 1")) -> (s? t:f=w540:string)
      n394 = local write "STATUS 1"(w540) -> ()
      "Done!" <- w535
    }
  }
